vi "Wago Input Voltage Monitor.vi"(8 "error in (no error)":errorcluster, 10 "Wago Data Input":T2 {"Input Process Image"."Software Constants"."Room PID Settings"."Room Dehumid Temperature I (*RM Dehum I1)" max=30000 step=1; "Input Process Image"."Software Constants"."Room PID Settings"."Room Dehumid Temperature P (*RM Dehum P1)" max=30000 step=1; "Input Process Image"."Software Constants"."Room PID Settings"."Room Cool Temperature I (*RM Cool I1)" max=30000 step=1; "Input Process Image"."Software Constants"."Room PID Settings"."Room Cool Temperature P (*RM Cool P1)" max=30000 step=1; "Input Process Image"."Software Constants"."Room PID Settings"."Room Heat I (*RM Heat I1)" max=30000 step=1; "Input Process Image"."Software Constants"."Room PID Settings"."Room Heat P (*RM Heat P1)" max=30000 step=1; "Input Process Image"."Software Constants"."Room PID Settings"."Room Humidity I (*RM Hum I1)" max=30000 step=1; "Input Process Image"."Software Constants"."Room PID Settings"."Room Humidity P (*RM Hum P1)" max=30000 step=1; "Input Process Image"."Software Constants"."Room PID Settings"."Room Dry I (*RM Dry I1)" max=30000 step=1; "Input Process Image"."Software Constants"."Room PID Settings"."Room Dry P(*RM Dry P1)" max=30000 step=1}, 11 "Modbus Master in":refnum<class "Modbus Master.lvclass">) -> (0 "error out (no error)":errorcluster, 2 "Wago Data Output":T2 {"Input Process Image"."Software Constants"."Room PID Settings"."Room Dehumid Temperature I (*RM Dehum I1)" max=30000 step=1; "Input Process Image"."Software Constants"."Room PID Settings"."Room Dehumid Temperature P (*RM Dehum P1)" max=30000 step=1; "Input Process Image"."Software Constants"."Room PID Settings"."Room Cool Temperature I (*RM Cool I1)" max=30000 step=1; "Input Process Image"."Software Constants"."Room PID Settings"."Room Cool Temperature P (*RM Cool P1)" max=30000 step=1; "Input Process Image"."Software Constants"."Room PID Settings"."Room Heat I (*RM Heat I1)" max=30000 step=1; "Input Process Image"."Software Constants"."Room PID Settings"."Room Heat P (*RM Heat P1)" max=30000 step=1; "Input Process Image"."Software Constants"."Room PID Settings"."Room Humidity I (*RM Hum I1)" max=30000 step=1; "Input Process Image"."Software Constants"."Room PID Settings"."Room Humidity P (*RM Hum P1)" max=30000 step=1; "Input Process Image"."Software Constants"."Room PID Settings"."Room Dry I (*RM Dry I1)" max=30000 step=1; "Input Process Image"."Software Constants"."Room PID Settings"."Room Dry P(*RM Dry P1)" max=30000 step=1}, 3 "Modbus master out":refnum<class "Modbus Master.lvclass">)   [LabVIEW 2016]
uses:
  <vilib>/NI/Modbus Library/API/Master/Modbus Master.lvclass
  Type Definitions/Wago Main Control.ctl
  Type Definitions/Wago Output Data Process Image.ctl
  Type Definitions/Wago Room Condtions.ctl
  Type Definitions/Wago Door Relays.ctl
  Type Definitions/Wago Contactor Settings.ctl
  Type Definitions/Wago Ground Leakage.ctl
  Type Definitions/Wago Input Process Image.ctl
  Type Definitions/Wago Room PID Settings.ctl
  Type Definitions/Wago Measured Input Data.ctl
  Type Definitions/Wago Room Setpoint Targets.ctl
  Type Definitions/Wago Output Commands.ctl
panel:
  in  "Wago Output Words 8":T1=791 items=["twHeatCtrl"=512, "twSteamCtrl"=513, "twCoolCtrl"=514, "twDehumCtrl"=515, "Output QX4 Bool"=516, "Output QX5 Bool"=517, "Output QX6 Bool"=518, "Output QX7 Bool"=519, "Output QX8 Bool"=520, "Output QX9 Bool"=521, "Output QX10"=522, "twRoomTemp"=840, "twRoomHum"=841, "twSuppTemp"=842, "twCoolTemp"=843, "twDehumTemp"=844, "twGlycolTemp"=845, "twHeatRate"=846, "twSteamRate"=847, "twCoolRate"=848, "twDehumRate"=849, "twStatus"=850, "twDoorEna"=851, "Rm1St1Dr1Stat"=816, "Rm1St2Dr1Stat"=817, "Rm1St3Dr1Stat"=818, "Rm1St4Dr1Stat"=819, "Rm1St5Dr1Stat"=820, "Rm1St6Dr1Stat"=821, "Rm1St7Dr1Stat"=822, "Rm1St8Dr1Stat"=823, "Rm1St1Dr2Stat"=824, "Rm1St2Dr2Stat"=825, "Rm1St3Dr2Stat"=826, "Rm1St4Dr2Stat"=827, "Rm1St5Dr2Stat"=828, "Rm1St6DrStat"=829, "Rm1St7Dr2Stat"=830, "Rm1St8Dr2Stat"=831, "Rm1St1Dr3Stat"=832, "Rm1St2Dr3Stat"=833, "Rm1St3Dr3Stat"=834, "Rm1St4Dr3Stat"=835, "Rm1St5Dr3Stat"=836, "Rm1St6Dr3Stat"=837, "Rm1St7Dr3Stat"=838, "Rm1St8Dr3Stat"=839, "twVoltMon1"=784, "twVoltMon2"=785, "twVoltMon3"=786, "twVoltMon4"=787, "twVoltMon5"=788, "twVoltMon6"=789, "twVoltMon7"=790, "twVoltMon8"=791, "twVoltStat1"=792, "twVoltStat2"=793, "twVoltStat3"=794, "twVoltStat4"=795, "twVoltStat5"=796, "twVoltStat6"=797, "twVoltStat7"=798, "twVoltStat8"=799]
  in  "Wago Output Words 7":T1=790 items=["twHeatCtrl"=512, "twSteamCtrl"=513, "twCoolCtrl"=514, "twDehumCtrl"=515, "Output QX4 Bool"=516, "Output QX5 Bool"=517, "Output QX6 Bool"=518, "Output QX7 Bool"=519, "Output QX8 Bool"=520, "Output QX9 Bool"=521, "Output QX10"=522, "twRoomTemp"=840, "twRoomHum"=841, "twSuppTemp"=842, "twCoolTemp"=843, "twDehumTemp"=844, "twGlycolTemp"=845, "twHeatRate"=846, "twSteamRate"=847, "twCoolRate"=848, "twDehumRate"=849, "twStatus"=850, "twDoorEna"=851, "Rm1St1Dr1Stat"=816, "Rm1St2Dr1Stat"=817, "Rm1St3Dr1Stat"=818, "Rm1St4Dr1Stat"=819, "Rm1St5Dr1Stat"=820, "Rm1St6Dr1Stat"=821, "Rm1St7Dr1Stat"=822, "Rm1St8Dr1Stat"=823, "Rm1St1Dr2Stat"=824, "Rm1St2Dr2Stat"=825, "Rm1St3Dr2Stat"=826, "Rm1St4Dr2Stat"=827, "Rm1St5Dr2Stat"=828, "Rm1St6DrStat"=829, "Rm1St7Dr2Stat"=830, "Rm1St8Dr2Stat"=831, "Rm1St1Dr3Stat"=832, "Rm1St2Dr3Stat"=833, "Rm1St3Dr3Stat"=834, "Rm1St4Dr3Stat"=835, "Rm1St5Dr3Stat"=836, "Rm1St6Dr3Stat"=837, "Rm1St7Dr3Stat"=838, "Rm1St8Dr3Stat"=839, "twVoltMon1"=784, "twVoltMon2"=785, "twVoltMon3"=786, "twVoltMon4"=787, "twVoltMon5"=788, "twVoltMon6"=789, "twVoltMon7"=790, "twVoltMon8"=791, "twVoltStat1"=792, "twVoltStat2"=793, "twVoltStat3"=794, "twVoltStat4"=795, "twVoltStat5"=796, "twVoltStat6"=797, "twVoltStat7"=798, "twVoltStat8"=799]
  in  "Wago Output Words 6":T1=789 items=["twHeatCtrl"=512, "twSteamCtrl"=513, "twCoolCtrl"=514, "twDehumCtrl"=515, "Output QX4 Bool"=516, "Output QX5 Bool"=517, "Output QX6 Bool"=518, "Output QX7 Bool"=519, "Output QX8 Bool"=520, "Output QX9 Bool"=521, "Output QX10"=522, "twRoomTemp"=840, "twRoomHum"=841, "twSuppTemp"=842, "twCoolTemp"=843, "twDehumTemp"=844, "twGlycolTemp"=845, "twHeatRate"=846, "twSteamRate"=847, "twCoolRate"=848, "twDehumRate"=849, "twStatus"=850, "twDoorEna"=851, "Rm1St1Dr1Stat"=816, "Rm1St2Dr1Stat"=817, "Rm1St3Dr1Stat"=818, "Rm1St4Dr1Stat"=819, "Rm1St5Dr1Stat"=820, "Rm1St6Dr1Stat"=821, "Rm1St7Dr1Stat"=822, "Rm1St8Dr1Stat"=823, "Rm1St1Dr2Stat"=824, "Rm1St2Dr2Stat"=825, "Rm1St3Dr2Stat"=826, "Rm1St4Dr2Stat"=827, "Rm1St5Dr2Stat"=828, "Rm1St6DrStat"=829, "Rm1St7Dr2Stat"=830, "Rm1St8Dr2Stat"=831, "Rm1St1Dr3Stat"=832, "Rm1St2Dr3Stat"=833, "Rm1St3Dr3Stat"=834, "Rm1St4Dr3Stat"=835, "Rm1St5Dr3Stat"=836, "Rm1St6Dr3Stat"=837, "Rm1St7Dr3Stat"=838, "Rm1St8Dr3Stat"=839, "twVoltMon1"=784, "twVoltMon2"=785, "twVoltMon3"=786, "twVoltMon4"=787, "twVoltMon5"=788, "twVoltMon6"=789, "twVoltMon7"=790, "twVoltMon8"=791, "twVoltStat1"=792, "twVoltStat2"=793, "twVoltStat3"=794, "twVoltStat4"=795, "twVoltStat5"=796, "twVoltStat6"=797, "twVoltStat7"=798, "twVoltStat8"=799]
  in  "Wago Output Words 5":T1=788 items=["twHeatCtrl"=512, "twSteamCtrl"=513, "twCoolCtrl"=514, "twDehumCtrl"=515, "Output QX4 Bool"=516, "Output QX5 Bool"=517, "Output QX6 Bool"=518, "Output QX7 Bool"=519, "Output QX8 Bool"=520, "Output QX9 Bool"=521, "Output QX10"=522, "twRoomTemp"=840, "twRoomHum"=841, "twSuppTemp"=842, "twCoolTemp"=843, "twDehumTemp"=844, "twGlycolTemp"=845, "twHeatRate"=846, "twSteamRate"=847, "twCoolRate"=848, "twDehumRate"=849, "twStatus"=850, "twDoorEna"=851, "Rm1St1Dr1Stat"=816, "Rm1St2Dr1Stat"=817, "Rm1St3Dr1Stat"=818, "Rm1St4Dr1Stat"=819, "Rm1St5Dr1Stat"=820, "Rm1St6Dr1Stat"=821, "Rm1St7Dr1Stat"=822, "Rm1St8Dr1Stat"=823, "Rm1St1Dr2Stat"=824, "Rm1St2Dr2Stat"=825, "Rm1St3Dr2Stat"=826, "Rm1St4Dr2Stat"=827, "Rm1St5Dr2Stat"=828, "Rm1St6DrStat"=829, "Rm1St7Dr2Stat"=830, "Rm1St8Dr2Stat"=831, "Rm1St1Dr3Stat"=832, "Rm1St2Dr3Stat"=833, "Rm1St3Dr3Stat"=834, "Rm1St4Dr3Stat"=835, "Rm1St5Dr3Stat"=836, "Rm1St6Dr3Stat"=837, "Rm1St7Dr3Stat"=838, "Rm1St8Dr3Stat"=839, "twVoltMon1"=784, "twVoltMon2"=785, "twVoltMon3"=786, "twVoltMon4"=787, "twVoltMon5"=788, "twVoltMon6"=789, "twVoltMon7"=790, "twVoltMon8"=791, "twVoltStat1"=792, "twVoltStat2"=793, "twVoltStat3"=794, "twVoltStat4"=795, "twVoltStat5"=796, "twVoltStat6"=797, "twVoltStat7"=798, "twVoltStat8"=799]
  in  "Wago Output Words 4":T1=787 items=["twHeatCtrl"=512, "twSteamCtrl"=513, "twCoolCtrl"=514, "twDehumCtrl"=515, "Output QX4 Bool"=516, "Output QX5 Bool"=517, "Output QX6 Bool"=518, "Output QX7 Bool"=519, "Output QX8 Bool"=520, "Output QX9 Bool"=521, "Output QX10"=522, "twRoomTemp"=840, "twRoomHum"=841, "twSuppTemp"=842, "twCoolTemp"=843, "twDehumTemp"=844, "twGlycolTemp"=845, "twHeatRate"=846, "twSteamRate"=847, "twCoolRate"=848, "twDehumRate"=849, "twStatus"=850, "twDoorEna"=851, "Rm1St1Dr1Stat"=816, "Rm1St2Dr1Stat"=817, "Rm1St3Dr1Stat"=818, "Rm1St4Dr1Stat"=819, "Rm1St5Dr1Stat"=820, "Rm1St6Dr1Stat"=821, "Rm1St7Dr1Stat"=822, "Rm1St8Dr1Stat"=823, "Rm1St1Dr2Stat"=824, "Rm1St2Dr2Stat"=825, "Rm1St3Dr2Stat"=826, "Rm1St4Dr2Stat"=827, "Rm1St5Dr2Stat"=828, "Rm1St6DrStat"=829, "Rm1St7Dr2Stat"=830, "Rm1St8Dr2Stat"=831, "Rm1St1Dr3Stat"=832, "Rm1St2Dr3Stat"=833, "Rm1St3Dr3Stat"=834, "Rm1St4Dr3Stat"=835, "Rm1St5Dr3Stat"=836, "Rm1St6Dr3Stat"=837, "Rm1St7Dr3Stat"=838, "Rm1St8Dr3Stat"=839, "twVoltMon1"=784, "twVoltMon2"=785, "twVoltMon3"=786, "twVoltMon4"=787, "twVoltMon5"=788, "twVoltMon6"=789, "twVoltMon7"=790, "twVoltMon8"=791, "twVoltStat1"=792, "twVoltStat2"=793, "twVoltStat3"=794, "twVoltStat4"=795, "twVoltStat5"=796, "twVoltStat6"=797, "twVoltStat7"=798, "twVoltStat8"=799]
  in  "Wago Output Words 3":T1=786 items=["twHeatCtrl"=512, "twSteamCtrl"=513, "twCoolCtrl"=514, "twDehumCtrl"=515, "Output QX4 Bool"=516, "Output QX5 Bool"=517, "Output QX6 Bool"=518, "Output QX7 Bool"=519, "Output QX8 Bool"=520, "Output QX9 Bool"=521, "Output QX10"=522, "twRoomTemp"=840, "twRoomHum"=841, "twSuppTemp"=842, "twCoolTemp"=843, "twDehumTemp"=844, "twGlycolTemp"=845, "twHeatRate"=846, "twSteamRate"=847, "twCoolRate"=848, "twDehumRate"=849, "twStatus"=850, "twDoorEna"=851, "Rm1St1Dr1Stat"=816, "Rm1St2Dr1Stat"=817, "Rm1St3Dr1Stat"=818, "Rm1St4Dr1Stat"=819, "Rm1St5Dr1Stat"=820, "Rm1St6Dr1Stat"=821, "Rm1St7Dr1Stat"=822, "Rm1St8Dr1Stat"=823, "Rm1St1Dr2Stat"=824, "Rm1St2Dr2Stat"=825, "Rm1St3Dr2Stat"=826, "Rm1St4Dr2Stat"=827, "Rm1St5Dr2Stat"=828, "Rm1St6DrStat"=829, "Rm1St7Dr2Stat"=830, "Rm1St8Dr2Stat"=831, "Rm1St1Dr3Stat"=832, "Rm1St2Dr3Stat"=833, "Rm1St3Dr3Stat"=834, "Rm1St4Dr3Stat"=835, "Rm1St5Dr3Stat"=836, "Rm1St6Dr3Stat"=837, "Rm1St7Dr3Stat"=838, "Rm1St8Dr3Stat"=839, "twVoltMon1"=784, "twVoltMon2"=785, "twVoltMon3"=786, "twVoltMon4"=787, "twVoltMon5"=788, "twVoltMon6"=789, "twVoltMon7"=790, "twVoltMon8"=791, "twVoltStat1"=792, "twVoltStat2"=793, "twVoltStat3"=794, "twVoltStat4"=795, "twVoltStat5"=796, "twVoltStat6"=797, "twVoltStat7"=798, "twVoltStat8"=799]
  in  "Wago Output Words 2":T1=785 items=["twHeatCtrl"=512, "twSteamCtrl"=513, "twCoolCtrl"=514, "twDehumCtrl"=515, "Output QX4 Bool"=516, "Output QX5 Bool"=517, "Output QX6 Bool"=518, "Output QX7 Bool"=519, "Output QX8 Bool"=520, "Output QX9 Bool"=521, "Output QX10"=522, "twRoomTemp"=840, "twRoomHum"=841, "twSuppTemp"=842, "twCoolTemp"=843, "twDehumTemp"=844, "twGlycolTemp"=845, "twHeatRate"=846, "twSteamRate"=847, "twCoolRate"=848, "twDehumRate"=849, "twStatus"=850, "twDoorEna"=851, "Rm1St1Dr1Stat"=816, "Rm1St2Dr1Stat"=817, "Rm1St3Dr1Stat"=818, "Rm1St4Dr1Stat"=819, "Rm1St5Dr1Stat"=820, "Rm1St6Dr1Stat"=821, "Rm1St7Dr1Stat"=822, "Rm1St8Dr1Stat"=823, "Rm1St1Dr2Stat"=824, "Rm1St2Dr2Stat"=825, "Rm1St3Dr2Stat"=826, "Rm1St4Dr2Stat"=827, "Rm1St5Dr2Stat"=828, "Rm1St6DrStat"=829, "Rm1St7Dr2Stat"=830, "Rm1St8Dr2Stat"=831, "Rm1St1Dr3Stat"=832, "Rm1St2Dr3Stat"=833, "Rm1St3Dr3Stat"=834, "Rm1St4Dr3Stat"=835, "Rm1St5Dr3Stat"=836, "Rm1St6Dr3Stat"=837, "Rm1St7Dr3Stat"=838, "Rm1St8Dr3Stat"=839, "twVoltMon1"=784, "twVoltMon2"=785, "twVoltMon3"=786, "twVoltMon4"=787, "twVoltMon5"=788, "twVoltMon6"=789, "twVoltMon7"=790, "twVoltMon8"=791, "twVoltStat1"=792, "twVoltStat2"=793, "twVoltStat3"=794, "twVoltStat4"=795, "twVoltStat5"=796, "twVoltStat6"=797, "twVoltStat7"=798, "twVoltStat8"=799]
  in  "Wago Output Words":T1=784 items=["twHeatCtrl"=512, "twSteamCtrl"=513, "twCoolCtrl"=514, "twDehumCtrl"=515, "Output QX4 Bool"=516, "Output QX5 Bool"=517, "Output QX6 Bool"=518, "Output QX7 Bool"=519, "Output QX8 Bool"=520, "Output QX9 Bool"=521, "Output QX10"=522, "twRoomTemp"=840, "twRoomHum"=841, "twSuppTemp"=842, "twCoolTemp"=843, "twDehumTemp"=844, "twGlycolTemp"=845, "twHeatRate"=846, "twSteamRate"=847, "twCoolRate"=848, "twDehumRate"=849, "twStatus"=850, "twDoorEna"=851, "Rm1St1Dr1Stat"=816, "Rm1St2Dr1Stat"=817, "Rm1St3Dr1Stat"=818, "Rm1St4Dr1Stat"=819, "Rm1St5Dr1Stat"=820, "Rm1St6Dr1Stat"=821, "Rm1St7Dr1Stat"=822, "Rm1St8Dr1Stat"=823, "Rm1St1Dr2Stat"=824, "Rm1St2Dr2Stat"=825, "Rm1St3Dr2Stat"=826, "Rm1St4Dr2Stat"=827, "Rm1St5Dr2Stat"=828, "Rm1St6DrStat"=829, "Rm1St7Dr2Stat"=830, "Rm1St8Dr2Stat"=831, "Rm1St1Dr3Stat"=832, "Rm1St2Dr3Stat"=833, "Rm1St3Dr3Stat"=834, "Rm1St4Dr3Stat"=835, "Rm1St5Dr3Stat"=836, "Rm1St6Dr3Stat"=837, "Rm1St7Dr3Stat"=838, "Rm1St8Dr3Stat"=839, "twVoltMon1"=784, "twVoltMon2"=785, "twVoltMon3"=786, "twVoltMon4"=787, "twVoltMon5"=788, "twVoltMon6"=789, "twVoltMon7"=790, "twVoltMon8"=791, "twVoltStat1"=792, "twVoltStat2"=793, "twVoltStat3"=794, "twVoltStat4"=795, "twVoltStat5"=796, "twVoltStat6"=797, "twVoltStat7"=798, "twVoltStat8"=799]
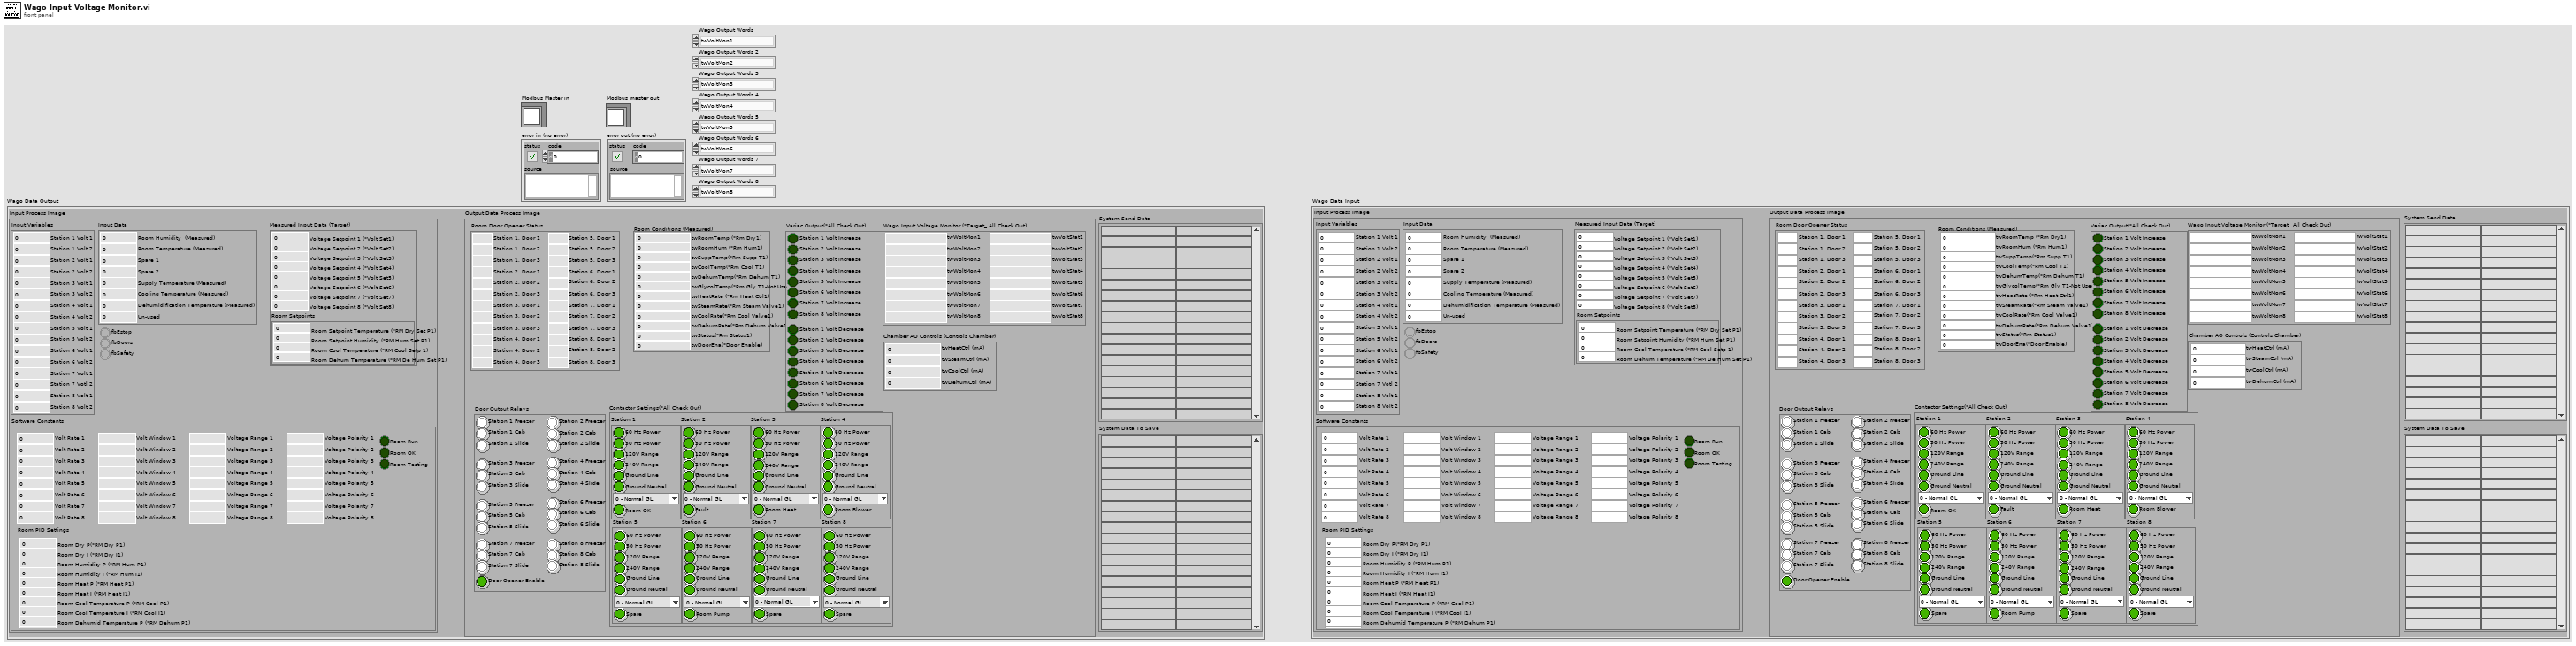
[diagram p1: front panel]
types:
  T1 = typedef "Wago Output Commands.ctl" = u16
  T2 = typedef "Wago Main Control.ctl" = cluster{"Output Data Process Image":T3, "Input Process Image":T8, "System Send Data":string[][], "System Data To Save":string[][]}
  T3 = typedef "Wago Output Data Process Image.ctl" = cluster{"Room Door Opener Status":cluster{"Station 1, Door 1":u16, "Station 1, Door 2":u16, "Station 1, Door 3":u16, "Station 2, Door 1":u16, "Station 2, Door 2":u16, "Station 2, Door 3":u16, "Station 3, Door 1":u16, "Station 3, Door 2":u16, "Station 3, Door 3":u16, "Station 4, Door 1":u16, "Station 4, Door 2":u16, "Station 4, Door 3":u16, "Station 5, Door 1":u16, "Station 5, Door 2":u16, "Station 5, Door 3":u16, "Station 6, Door 1":u16, "Station 6, Door 2":u16, "Station 6, Door 3":u16, "Station 7, Door 1":u16, "Station 7, Door 2":u16, "Station 7, Door 3":u16, "Station 8, Door 1":u16, "Station 8, Door 2":u16, "Station 8, Door 3":u16}, "Room Conditions (Measured)":T4, "Chamber AO Controls (Controls Chamber)":cluster{"twDehumCtrl (mA)":u16, "twCoolCtrl (mA)":u16, "twSteamCtrl (mA)":u16, "twHeatCtrl (mA)":u16}, "Variac Output(*All Check Out)":cluster{"Station 1 Volt Increase":bool, "Station 1 Volt Decrease":bool, "Station 2 Volt Increase":bool, "Station 2 Volt Decrease":bool, "Station 3 Volt Increase":bool, "Station 3 Volt Decrease":bool, "Station 4 Volt Increase":bool, "Station 4 Volt Decrease":bool, "Station 5 Volt Increase":bool, "Station 5 Volt Decrease":bool, "Station 6 Volt Increase":bool, "Station 6 Volt Decrease":bool, "Station 7 Volt Increase":bool, "Station 7 Volt Decrease":bool, "Station 8 Volt Increase":bool, "Station 8 Volt Decrease":bool}, "Door Output Relays":T5, "Wago Input Voltage Monitor (*Target_ All Check Out)":cluster{"twWoltMon1":dbl, "twWoltMon2":dbl, "twWoltMon3":dbl, "twWoltMon4":dbl, "twWoltMon5":dbl, "twWoltMon6":dbl, "twWoltMon7":dbl, "twWoltMon8":dbl, "twVoltStat1":u16, "twVoltStat2":u16, "twVoltStat3":u16, "twVoltStat4":u16, "twVoltStat5":u16, "twVoltStat6":u16, "twVoltStat7":u16, "twVoltStat8":u16}, "Contactor Settings(*All Check Out)":T6}
  T4 = typedef "Wago Room Condtions.ctl" = cluster{"twDoorEna(*Door Enable)":u16, "twStatus(*Rm Status1)":u16, "twRoomTemp (*Rm Dry1)":dbl, "twRoomHum (*Rm Hum1)":dbl, "twSuppTemp(*Rm Supp T1)":dbl, "twCoolTemp(*Rm Cool T1)":dbl, "twDehumTemp(*Rm Dehum T1)":dbl, "twGlycolTemp(*Rm Gly T1-Not Used)":dbl, "twDehumRate(*Rm Dehum Valve1)":dbl, "twCoolRate(*Rm Cool Valve1)":dbl, "twSteamRate(*Rm Steam Valve1)":dbl, "twHeatRate (*Rm Heat Ctrl1)":dbl}
  T5 = typedef "Wago Door Relays.ctl" = cluster{"Station 1 Freezer":bool, "Station 1 Cab":bool, "Station 1 Slide":bool, "Station 2 Freezer":bool, "Station 2 Cab":bool, "Station 2 Slide":bool, "Station 3 Freezer":bool, "Station 3 Cab":bool, "Station 3 Slide":bool, "Station 4 Freezer":bool, "Station 4 Cab":bool, "Station 4 Slide":bool, "Station 5 Freezer":bool, "Station 5 Cab":bool, "Station 5 Slide":bool, "Station 6 Freezer":bool, "Station 6 Cab":bool, "Station 6 Slide":bool, "Station 7 Freezer":bool, "Station 7 Cab":bool, "Station 7 Slide":bool, "Station 8 Freezer":bool, "Station 8 Cab":bool, "Station 8 Slide":bool, "Door Opener Enable":bool}
  T6 = typedef "Wago Contactor Settings.ctl" = cluster{"Station 1":cluster{"60 Hz Power":bool, "50 Hz Power":bool, "120V Range":bool, "240V Range":bool, "Ground Line":bool, "Ground Neutral":bool, "Room OK":bool, "Ground Leakage":T7}, "Station 2":cluster{"60 Hz Power":bool, "50 Hz Power":bool, "120V Range":bool, "240V Range":bool, "Ground Line":bool, "Ground Neutral":bool, "Fault":bool, "Ground Leakage":T7}, "Station 3":cluster{"60 Hz Power":bool, "50 Hz Power":bool, "120V Range":bool, "240V Range":bool, "Ground Line":bool, "Ground Neutral":bool, "Room Heat":bool, "Ground Leakage":T7}, "Station 4":cluster{"60 Hz Power":bool, "50 Hz Power":bool, "120V Range":bool, "240V Range":bool, "Ground Line":bool, "Ground Neutral":bool, "Room Blower":bool, "Ground Leakage":T7}, "Station 5":cluster{"60 Hz Power":bool, "50 Hz Power":bool, "120V Range":bool, "240V Range":bool, "Ground Line":bool, "Ground Neutral":bool, "Spare":bool, "Ground Leakage":T7}, "Station 6":cluster{"60 Hz Power":bool, "50 Hz Power":bool, "120V Range":bool, "240V Range":bool, "Ground Line":bool, "Ground Neutral":bool, "Room Pump":bool, "Ground Leakage":T7}, "Station 7":cluster{"60 Hz Power":bool, "50 Hz Power":bool, "120V Range":bool, "240V Range":bool, "Ground Line":bool, "Ground Neutral":bool, "Spare":bool, "Ground Leakage":T7}, "Station 8":cluster{"60 Hz Power":bool, "50 Hz Power":bool, "120V Range":bool, "240V Range":bool, "Ground Line":bool, "Ground Neutral":bool, "Spare":bool, "Ground Leakage":T7}}
  T7 = typedef "Wago Ground Leakage.ctl" = enum16{"0 - Normal GL", "1 - Measure GL"}
  T8 = typedef "Wago Input Process Image.ctl" = cluster{"fbEstop":bool, "fbDoors":bool, "fbSafety":bool, "Input Variables":cluster{"Station 1 Volt 1":dbl, "Station 1 Volt 2":dbl, "Station 2 Volt 1":dbl, "Station 2 Volt 2":dbl, "Station 3 Volt 1":dbl, "Station 3 Volt 2":dbl, "Station 4 Volt 1":dbl, "Station 4 Volt 2":dbl, "Station 5 Volt 1":dbl, "Station 5 Volt 2":dbl, "Station 6 Volt 1":dbl, "Station 6 Volt 2":dbl, "Station 7 Volt 1":dbl, "Station 7 Votl 2":dbl, "Station 8 Volt 1":dbl, "Station 8 Volt 2":dbl}, "Input Data":cluster{"Room Humidity  (Measured)":dbl, "Room Temperature (Measured)":dbl, "Spare 1":dbl, "Spare 2":dbl, "Supply Temperature (Measured)":dbl, "Cooling Temperature (Measured)":dbl, "Dehumidification Temperature (Measured)":dbl, "Un-used":dbl}, "Software Constants":cluster{"Volt Rate 1":u16, "Volt Rate 2":u16, "Volt Rate 3":u16, "Volt Rate 4":u16, "Volt Rate 5":u16, "Volt Rate 6":u16, "Volt Rate 7":u16, "Volt Rate 8":u16, "Volt Window 1":u16, "Volt Window 2":u16, "Volt Window 3":u16, "Volt Window 4":u16, "Volt Window 5":u16, "Volt Window 6":u16, "Volt Window 7":u16, "Volt Window 8":u16, "Voltage Range 1":u16, "Voltage Range 2":u16, "Voltage Range 3":u16, "Voltage Range 4":u16, "Voltage Range 5":u16, "Voltage Range 6":u16, "Voltage Range 7":u16, "Voltage Range 8":u16, "Voltage Polarity 1":u16, "Voltage Polarity 2":u16, "Voltage Polarity 3":u16, "Voltage Polarity 4":u16, "Voltage Polarity 5":u16, "Voltage Polarity 6":u16, "Voltage Polarity 7":u16, "Voltage Polarity 8":u16, "Room Run":bool, "Room OK":bool, "Room Testing":bool, "Room PID Settings":T9}, "Measured Input Data (Target)":T10}
  T9 = typedef "Wago Room PID Settings.ctl" = cluster{"Room Dry P(*RM Dry P1)":u16, "Room Dry I (*RM Dry I1)":u16, "Room Humidity P (*RM Hum P1)":u16, "Room Humidity I (*RM Hum I1)":u16, "Room Heat P (*RM Heat P1)":u16, "Room Heat I (*RM Heat I1)":u16, "Room Cool Temperature P (*RM Cool P1)":u16, "Room Cool Temperature I (*RM Cool I1)":u16, "Room Dehumid Temperature P (*RM Dehum P1)":u16, "Room Dehumid Temperature I (*RM Dehum I1)":u16}
  T10 = typedef "Wago Measured Input Data.ctl" = cluster{"Voltage Setpoint 1 (*Volt Set1)":dbl, "Voltage Setpoint 2 (*Volt Set2)":dbl, "Voltage Setpoint 3 (*Volt Set3)":dbl, "Voltage Setpoint 4 (*Volt Set4)":dbl, "Voltage Setpoint 5 (*Volt Set5)":dbl, "Voltage Setpoint 6 (*Volt Set6)":dbl, "Voltage Setpoint 7 (*Volt Set7)":dbl, "Voltage Setpoint 8 (*Volt Set8)":dbl, "Room Setpoints":T11}
  T11 = typedef "Wago Room Setpoint Targets.ctl" = cluster{"Room Setpoint Temperature (*RM Dry Set P1)":dbl, "Room Setpoint Humidity (*RM Hum Set P1)":dbl, "Room Cool Temperature (*RM Cool Setp 1)":dbl, "Room Dehum Temperature (*RM De Hum Set P1)":dbl}
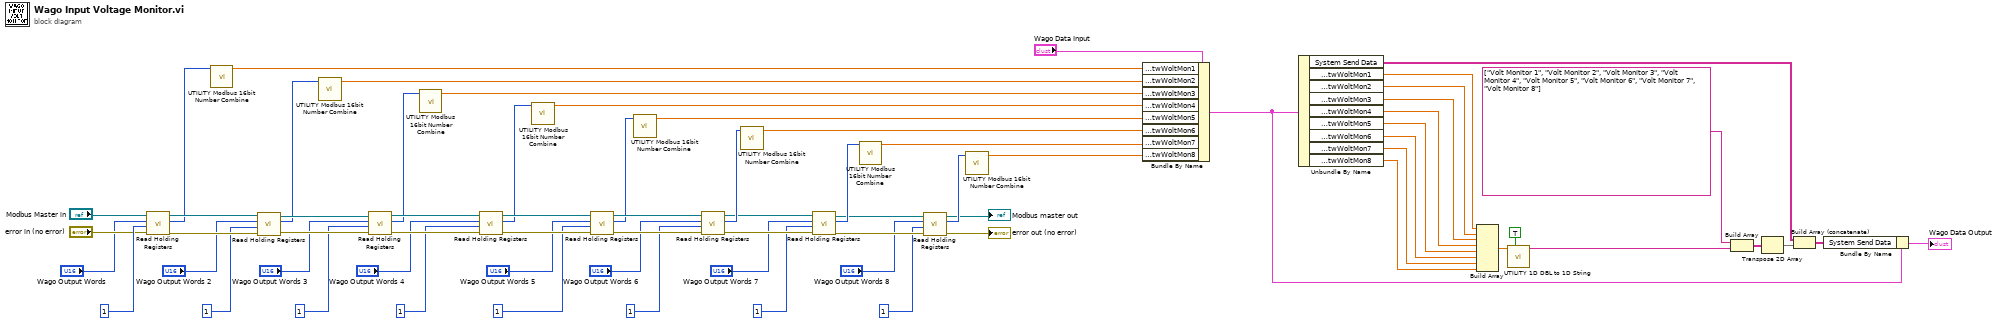
[diagram p0: block diagram]
diagram:
  n1 = call-dynamic "Read Holding Registers.vi"("error in"="error in (no error)", "number of inputs"=u16 1, "starting address"="Wago Output Words", "Modbus master in"="Modbus Master in") -> ("error out"=w50:errorcluster, "register values"=w40:u16[], "Modbus master out"=w51:refnum<class "Modbus Master.lvclass">)  [unwired: 5 in]
  n2 = call "UTILITY Modbus 16bit Number Combine.vi"("Holding Registers"=w40) -> ("Data"=w34:dbl)  [unwired: 10 in]
  n3 = call-dynamic "Read Holding Registers.vi"("error in"=w50, "number of inputs"=u16 1, "starting address"="Wago Output Words 2", "Modbus master in"=w51) -> ("error out"=w53:errorcluster, "register values"=w43:u16[], "Modbus master out"=w52:refnum<class "Modbus Master.lvclass">)  [unwired: 5 in]
  n4 = call "UTILITY Modbus 16bit Number Combine.vi"("Holding Registers"=w43) -> ("Data"=w33:dbl)  [unwired: 10 in]
  n5 = call-dynamic "Read Holding Registers.vi"("error in"=w53, "number of inputs"=u16 1, "starting address"="Wago Output Words 3", "Modbus master in"=w52) -> ("error out"=w55:errorcluster, "register values"=w44:u16[], "Modbus master out"=w54:refnum<class "Modbus Master.lvclass">)  [unwired: 5 in]
  n6 = call "UTILITY Modbus 16bit Number Combine.vi"("Holding Registers"=w44) -> ("Data"=w32:dbl)  [unwired: 10 in]
  n7 = call-dynamic "Read Holding Registers.vi"("error in"=w55, "number of inputs"=u16 1, "starting address"="Wago Output Words 4", "Modbus master in"=w54) -> ("error out"=w57:errorcluster, "register values"=w47:u16[], "Modbus master out"=w56:refnum<class "Modbus Master.lvclass">)  [unwired: 5 in]
  n8 = call "UTILITY Modbus 16bit Number Combine.vi"("Holding Registers"=w47) -> ("Data"=w31:dbl)  [unwired: 10 in]
  n9 = call-dynamic "Read Holding Registers.vi"("error in"=w57, "number of inputs"=u16 1, "starting address"="Wago Output Words 5", "Modbus master in"=w56) -> ("error out"=w61:errorcluster, "register values"=w48:u16[], "Modbus master out"=w62:refnum<class "Modbus Master.lvclass">)  [unwired: 5 in]
  n10 = call "UTILITY Modbus 16bit Number Combine.vi"("Holding Registers"=w48) -> ("Data"=w30:dbl)  [unwired: 10 in]
  n11 = call-dynamic "Read Holding Registers.vi"("error in"=w61, "number of inputs"=u16 1, "starting address"="Wago Output Words 6", "Modbus master in"=w62) -> ("error out"=w64:errorcluster, "register values"=w69:u16[], "Modbus master out"=w63:refnum<class "Modbus Master.lvclass">)  [unwired: 5 in]
  n12 = call "UTILITY Modbus 16bit Number Combine.vi"("Holding Registers"=w69) -> ("Data"=w29:dbl)  [unwired: 10 in]
  n13 = call-dynamic "Read Holding Registers.vi"("error in"=w64, "number of inputs"=u16 1, "starting address"="Wago Output Words 7", "Modbus master in"=w63) -> ("error out"=w66:errorcluster, "register values"=w68:u16[], "Modbus master out"=w65:refnum<class "Modbus Master.lvclass">)  [unwired: 5 in]
  n14 = call "UTILITY Modbus 16bit Number Combine.vi"("Holding Registers"=w68) -> ("Data"=w28:dbl)  [unwired: 10 in]
  n15 = call-dynamic "Read Holding Registers.vi"("error in"=w66, "number of inputs"=u16 1, "starting address"="Wago Output Words 8", "Modbus master in"=w65) -> ("error out"=→"error out (no error)":errorcluster, "register values"=w67:u16[], "Modbus master out"=→"Modbus master out":refnum<class "Modbus Master.lvclass">)  [unwired: 5 in]
  n16 = call "UTILITY Modbus 16bit Number Combine.vi"("Holding Registers"=w67) -> ("Data"=w27:dbl)  [unwired: 10 in]
  n17 = Bundle By Name(cluster="Wago Data Input", "Output Data Process Image.Wago Input Voltage Monitor (*Target_ All Check Out).twWoltMon1"=w34, "Output Data Process Image.Wago Input Voltage Monitor (*Target_ All Check Out).twWoltMon2"=w33, "Output Data Process Image.Wago Input Voltage Monitor (*Target_ All Check Out).twWoltMon3"=w32, "Output Data Process Image.Wago Input Voltage Monitor (*Target_ All Check Out).twWoltMon4"=w31, "Output Data Process Image.Wago Input Voltage Monitor (*Target_ All Check Out).twWoltMon5"=w30, "Output Data Process Image.Wago Input Voltage Monitor (*Target_ All Check Out).twWoltMon6"=w29, "Output Data Process Image.Wago Input Voltage Monitor (*Target_ All Check Out).twWoltMon7"=w28, "Output Data Process Image.Wago Input Voltage Monitor (*Target_ All Check Out).twWoltMon8"=w27) -> (w8:T2)
  n18 = Unbundle By Name(w8) -> ("System Send Data"=w12:string[][], "Output Data Process Image.Wago Input Voltage Monitor (*Target_ All Check Out).twWoltMon1"=w17:dbl, "Output Data Process Image.Wago Input Voltage Monitor (*Target_ All Check Out).twWoltMon2"=w7:dbl, "Output Data Process Image.Wago Input Voltage Monitor (*Target_ All Check Out).twWoltMon3"=w6:dbl, "Output Data Process Image.Wago Input Voltage Monitor (*Target_ All Check Out).twWoltMon4"=w5:dbl, "Output Data Process Image.Wago Input Voltage Monitor (*Target_ All Check Out).twWoltMon5"=w4:dbl, "Output Data Process Image.Wago Input Voltage Monitor (*Target_ All Check Out).twWoltMon6"=w3:dbl, "Output Data Process Image.Wago Input Voltage Monitor (*Target_ All Check Out).twWoltMon7"=w2:dbl, "Output Data Process Image.Wago Input Voltage Monitor (*Target_ All Check Out).twWoltMon8"=w1:dbl)
  n19 = Build Array(w17, w7, w6, w5, w4, w3, w2, w1) -> (w16:dbl[])
  n20 = call "UTILITY 1D DBL to 1D String.vi"("DBL?"=TRUE, "1D DBL"=w16) -> ("1D String"=w14:string[])  [unwired: 9 in]
  n21 = Build Array(string[] ["Volt Monitor 1", "Volt Monitor 2", "Volt Monitor 3", "Volt Monitor 4", "Volt Monitor 5", "Volt Monitor 6", "Volt Monitor 7", "Volt Monitor 8"], w14) -> (w13:string[][])
  n22 = Transpose 2D Array(2D array=w13) -> (transposed array=w11:string[][])
  n23 = Build Array (concatenate)(w12, w11) -> (w10:string[][])
  n24 = Bundle By Name(cluster=w8, "System Send Data"=w10) -> (→"Wago Data Output":T2)
